vi "PN Visible.vi"(8 "error in":errorcluster, 9 "Visible":bool, 11 "reference":refnum<vi>) -> (0 "error out":errorcluster)   [LabVIEW 2022 SP3]
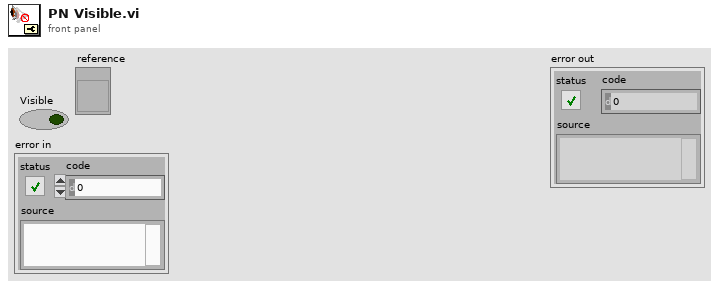
[diagram p1: front panel]
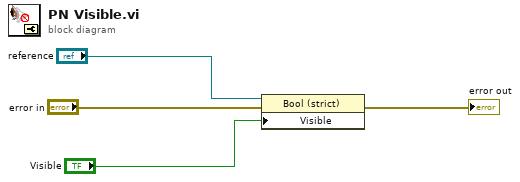
[diagram p0: block diagram]
diagram:
  n1 = property class="Bool (strict)"(reference="reference", error in="error in", "Visible"="Visible") -> (error out=→"error out":errorcluster)  [unwired: 1 out]
